vi "Get settings chain.vi"(8 "error in (no error)":errorcluster, 11 "ThorcamBase in":refnum<class "Thorcam.lvclass">) -> (0 "error out":errorcluster, 1 "class name":string[](array[string]), 2 "settings":variant[](array[variant]), 3 "ThorcamBase out":refnum<class "Thorcam.lvclass">)   [LabVIEW 2012, in "Thorcam.lvclass"]
doc: "Returns an array of variants containing the settings clusters of each class in the inheritance chain (lowest child class first), together with an array of all class names in the inheritance chain.\n\nFor classes without settings cluster, the settings chain contains empty variants."
uses:
  Thorcam.lvclass
  <vilib>/Distrio/Murmex/Murmex/Murmex.lvclass
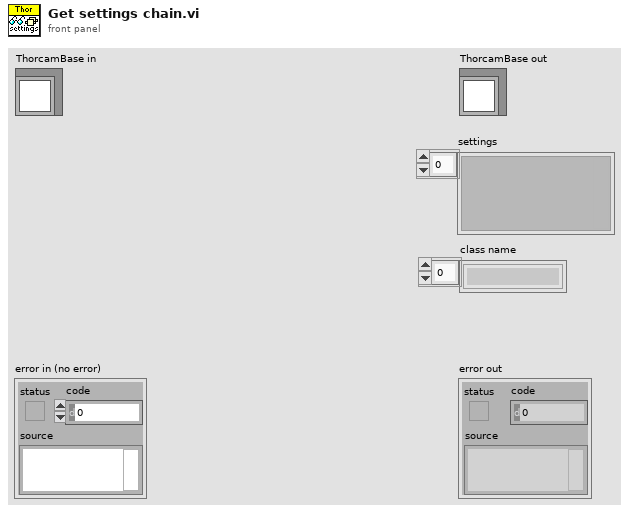
[diagram p1: front panel]
types:
  T1 = typedef "Thorcam.lvclass/settings.ctl" = cluster{"image":T2, "Pre-Tomo":T3, "Imaging mode":T4, "Camera settings":T5, "cross correlation":T6, "Filename":string, "Feed":T7}
  T2 = typedef "Thorcam.lvclass/image.ctl" = cluster{"gamma":i32, "offset":i32, "gain":i32, "hot pixel correction":bool}
  T3 = typedef "Thorcam.lvclass/pretomo.ctl" = cluster{"z-step":dbl[unit], "current_stack_x":dbl[unit], "current_stack_y":dbl[unit], "current_stack_z1":dbl[unit], "current_stack_z2":dbl[unit], "pre-tomo":bool, "number of frames":i32}
  T4 = typedef "Thorcam.lvclass/imaging mode.ctl" = enum16{"free run mode", "single frame"}
  T5 = typedef "Thorcam.lvclass/camera settings.ctl" = cluster{"exposure time ":dbl[unit], "frames per second":dbl, "pixel clock":dbl[unit]}
  T6 = typedef "Thorcam.lvclass/cross correlation settings.ctl" = cluster{"phase comparison interval":dbl[unit], "phase comparison threshold":dbl}
  T7 = typedef "Thorcam.lvclass/feed.ctl" = enum16{"Video", "Cross Correlation", "Rob and Roy", "Roy", "Rob"}
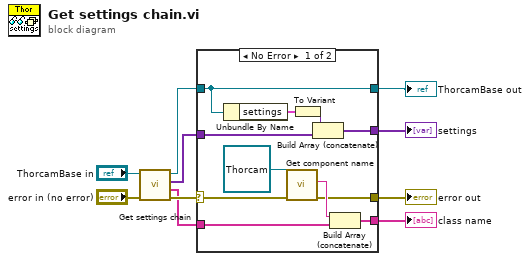
[diagram p0: block diagram]
diagram:
  n1 = call-parent "Get settings chain.vi"("error in (no error)"="error in (no error)", "MurmexBase in"="ThorcamBase in") -> ("error out"=w8:errorcluster, "class name"=w7:string[], "settings"=w3:variant[], "MurmexBase out"=w5:refnum<class "Thorcam.lvclass">)  [unwired: 6 in]
  n2 = case shown="No Error" w8 {
    selector: w8 -> [w18 w22]
    tunnel: w7 -> [w17 _]
    tunnel: [w16 w22] -> w6
    tunnel: w5 -> [w14 w23]
    tunnel: [w14 w23] -> w4
    tunnel: w3 -> [w13 _]
    tunnel: [w12 _] -> w2
    tunnel: [w11 _] -> w1
    frame No Error {
      n3 = Unbundle By Name(w14) -> ("settings"=w21:T1)
      n4 = call <vilib>:"Get component name.vi"("error in (no error)"=w18, "Murmex in"=refnum<class "Thorcam.lvclass"> refnum ("Thorcam")) -> ("error out"=w16:errorcluster, "component name"=w19:string)  [unwired: 7 in, 1 out]
      n5 = To Variant(anything=w21) -> (Variant=w20:variant)
      n6 = Build Array (concatenate)(w20, w13) -> (w12:variant[])
      n7 = Build Array (concatenate)(w19, w17) -> (w11:string[])
    }
    frame Error {
    }
  }
  "error out" <- w6
  "ThorcamBase out" <- w4
  "settings" <- w2
  "class name" <- w1
